vi "LCC Get Sw Scaling Param.vi"(8 "error in (no error)":errorcluster caption="Fehler (Eingang, kein Fehler)", 11 "Channel Handle":i64) -> (0 "error out":errorcluster caption="Fehler (Ausgang)", 2 "Scaling Offset":dbl, 3 "Scaling Factor":dbl)   [LabVIEW 2021, in "labbCAN_Controller_API.lvlib"]
doc: "LCC_Func long LCC_CALL LCC_GetSwScalingParam(dev_hdl ChanHdl,\n double *pfScalingFactor,\n double *pfScalingOffset);"
uses:
  labbCAN_Controller_API.lvlib
  labbCAN_Controller_API.dll
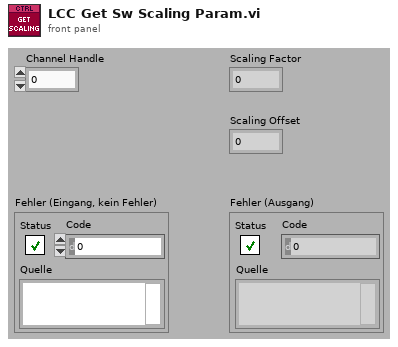
[diagram p1: front panel]
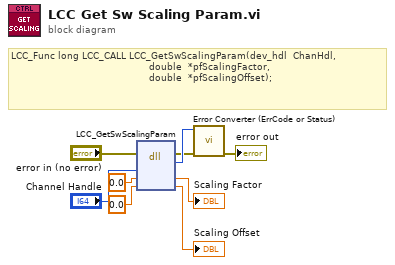
[diagram p0: block diagram]
diagram:
  # "LCC_Func long LCC_CALL LCC_GetSwScalingParam(dev_hdl  ChanHdl,\n                                              double  *pfScalingFactor,\n                                              double  *pfScalingOffset);"
  n1 = dll-call lib="C:/Users/olaja/AppData/Local/CETONI_SDK/labbCAN_Controller_API.*" fn="LCC_GetSwScalingParam"(error in="error in (no error)", "ChanHdl"="Channel Handle", "pfScalingFactor"=0.0, "pfScalingOffset"=0.0) -> (error out=w2:errorcluster, "Rückgabetyp"=w3:i32, "pfScalingFactor"=→"Scaling Factor":dbl, "pfScalingOffset"=→"Scaling Offset":dbl)  [unwired: 3 in, 1 out]
  n2 = call "Error Converter (ErrCode or Status).vi"("error in (no error)"=w2, "error code"=w3) -> ("error out"=→"error out":errorcluster)  [unwired: 9 in]
